vi "Example 1.vi"() -> ()   [LabVIEW 2014, in "UI_ProgressDlg.lvlib"]
uses:
  UI_ProgressDlg.lvlib
  _Control/DEF-Type.ctl
  UI_ProgressDlg.lvclass
panel:
  out "Stop TimeStamp":timestamp
  in  "Closeable?":bool=TRUE
  in  "Type":T1=enum."Timer Window"
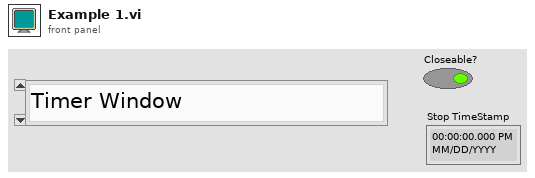
[diagram p1: front panel]
types:
  T1 = typedef "UI_ProgressDlg.lvlib/UI_ProgressDlg.lvclass/DEF-Type.ctl" = enum16{"Progress Window", "Buzy Window", "Timer Window"}
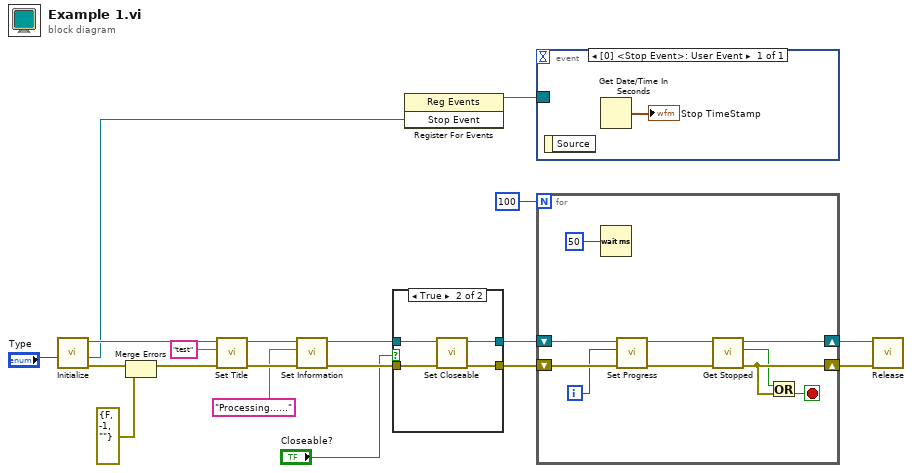
[diagram p0: block diagram]
diagram:
  n1 = call "Initialize.vi"("Type"="Type") -> ("error out"=w1:errorcluster, "Stop Event"=w3:refnum<user-event>, "UI_ProgressBar out"=w19:refnum<class "UI_ProgressDlg.lvclass">)  [unwired: 8 in]
  n2 = Merge Errors(w1, errorcluster {"status"=FALSE, "code"=-1, "source"=""} ("error in")) -> (w9:errorcluster)
  n3 = call "Set Title.vi"("error in (no error)"=w9, "title"="test", "UI_ProgressBar in"=w19) -> ("error out"=w16:errorcluster, "UI_ProgressBar out"=w17:refnum<class "UI_ProgressDlg.lvclass">)  [unwired: 7 in]
  n4 = call "Set Information.vi"("error in (no error)"=w16, "Inforamtion"="Processing......", "UI_ProgressBar in"=w17) -> ("error out"=w6:errorcluster, "UI_ProgressBar out"=w14:refnum<class "UI_ProgressDlg.lvclass">)  [unwired: 7 in]
  n5 = case shown="True" "Closeable?" {
    tunnel: w14 -> [w21 w25]
    tunnel: [w21 w24] -> w7
    tunnel: w6 -> [w20 w23]
    tunnel: [w20 w22] -> w5
    frame False {
    }
    frame True {
      n6 = call "Set Closeable.vi"("error in (no error)"=w23, "UI_ProgressBar in"=w25) -> ("error out"=w22:errorcluster, "UI_ProgressBar out"=w24:refnum<class "UI_ProgressDlg.lvclass">)  [unwired: 8 in]
    }
  }
  n7 = register-events(w3) -> (reference out=w2:refnum<event-registration>)  [unwired: 2 in, 1 out]
  n8 = event shown="[0] <Stop Event>: User Event" {
    selector: w2 -> [_]
    dyn-events: _ -> [_]
    timeout: _ -> [_]
    event User Event {
      n9 = event-data() -> ()  [unwired: 1 in, 1 out]
      n10 = Get Date/Time In Seconds() -> (seconds since 1Jan1904=→"Stop TimeStamp":timestamp)
    }
  }
  n11 = for {
    N: 100 -> [_]
    shift-right: [w32] -> w13
    shift-left: w7 -> [w36]
    shift-right: [w31] -> w12
    shift-left: w5 -> [w35]
    i -> [w34]
    stop <- w30 stop-if-true
    n12 = Wait (ms)(milliseconds to wait=u32 50) -> ()  [unwired: 1 out]
    n13 = call "Set Progress.vi"("error in (no error)"=w35, "progress"=w34, "UI_ProgressBar in"=w36) -> ("error out"=w28:errorcluster, "UI_ProgressBar out"=w27:refnum<class "UI_ProgressDlg.lvclass">)  [unwired: 7 in]
    n14 = call "Get Stopped.vi"("error in (no error)"=w28, "UI_ProgressDlg in"=w27) -> ("error out"=w31:errorcluster, "Stopped?"=w29:bool, "UI_ProgressDlg out"=w32:refnum<class "UI_ProgressDlg.lvclass">)  [unwired: 7 in]
    n15 = Or(x=w29, y=w31) -> (x .or. y?=w30:bool)
  }
  n16 = call "Release.vi"("error in (no error)"=w12, "UI_ProgressBar in"=w13) -> ()  [unwired: 8 in, 2 out]
